vi "Create.vi"(8 "error in (no error)":errorcluster) -> (0 "error out":errorcluster, 3 "Mock Class Generator out":refnum<class "Mock I2C Bus.lvclass">)   [LabVIEW 2020, in "Mock I2C Bus.lvclass"]
uses:
  Mock I2C Bus.lvclass
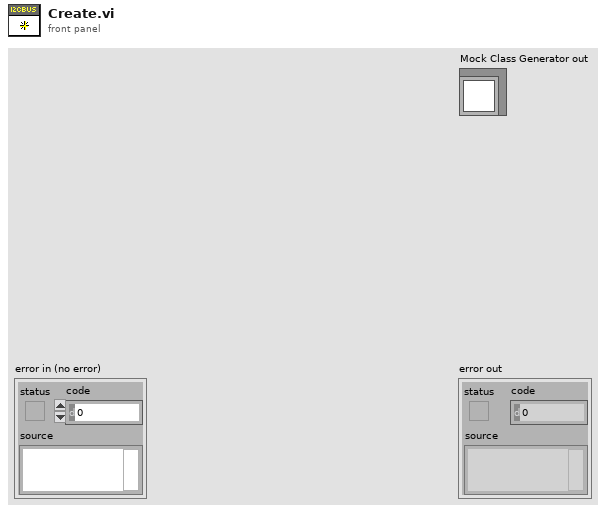
[diagram p1: front panel]
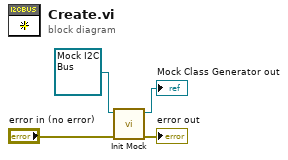
[diagram p0: block diagram]
diagram:
  n1 = call-dynamic "Init Mock.vi"("error in (no error)"="error in (no error)", "Mock In"=refnum<class "Mock I2C Bus.lvclass"> refnum ("Mock in")) -> ("error out"=→"error out":errorcluster, "Mock Out"=→"Mock Class Generator out":refnum<class "Mock I2C Bus.lvclass">)  [unwired: 8 in]
